vi "FIR Filter.vi"   [LabVIEW 2012, in "NI_AALBase.lvlib"]
doc: "Filters the input sequence<B> X</B> using the direct-form FIR filter specified by <B>FIR Coefficients</B>. Wire data to the <B>X</B> input to determine the polymorphic instance to use or manually select the instance."
uses:
  NI_AALBase.lvlib
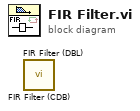
[diagram p0: block diagram]
diagram:
  n1 = call "FIR Filter (CDB).vi"() -> ()  [unwired: 4 in, 2 out]
  n2 = call "FIR Filter (DBL).vi"() -> ()  [unwired: 4 in, 2 out]
